vi "LVObject to JSON.vi"(5 "enable LabVIEW extensions? (T)":bool=TRUE, 6 "Pretty Print?":bool, 7 "Theme Serializer in":refnum<class "Theme Serializer.lvclass">, 8 "error in":errorcluster, 10 "Object":refnum<class>) -> (0 "error out":errorcluster, 2 "<JSON>Object":string)   [LabVIEW 2021, in "Theme Serializer.lvclass"]
doc: "Convert Object of a LabVIEW Class to a JSON representation."
uses:
  Theme Serializer.lvclass
  Theme Config/Theme Config.lvclass
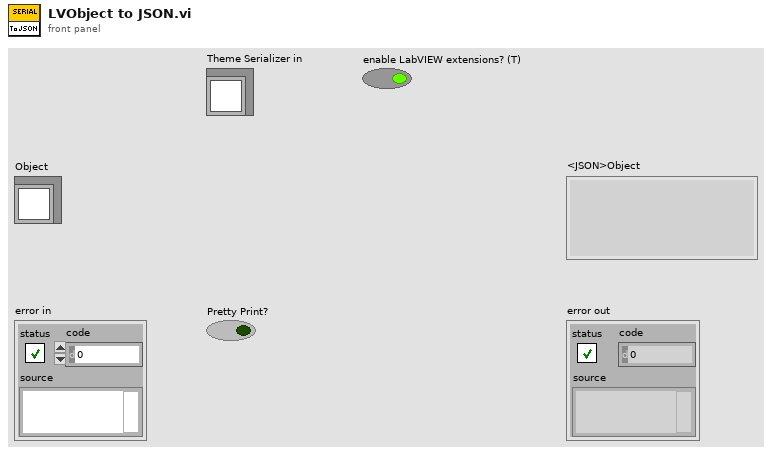
[diagram p1: front panel]
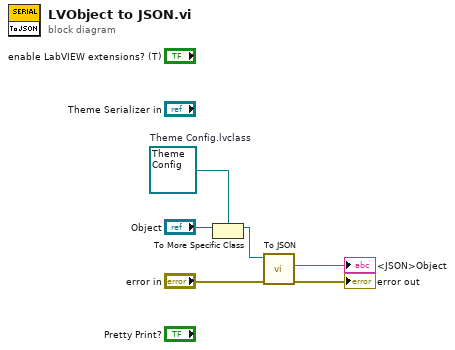
[diagram p0: block diagram]
diagram:
  w5 = refnum<class "Theme Config.lvclass"> refnum  # Theme Config.lvclass
  n1 = To More Specific Class(target class=w5, reference="Object") -> (specific class reference=w4:refnum<class "Theme Config.lvclass">)  [unwired: 1 in, 1 out]
  n2 = call "To JSON.vi"("error in"="error in", "Theme Config in"=w4) -> ("error out"=→"error out":errorcluster, "JSON"=→"<JSON>Object":string)  [unwired: 7 in, 1 out]
